vi "Setup.vi"(11 "error in":errorcluster) -> (4 "Application Ref":refnum<vi>, 6 "VI Reference Out":refnum<vi>, 15 "error out":errorcluster)   [LabVIEW 2016, in "Drona.lvlib"]
uses:
  Drona.lvlib
  _Typedefs/SetupSourceConfig.ctl
  _Typedefs/SetupEXEConfig.ctl
  GetVI/GetVIByPath.vi
  GetVI/GetVIByName.vi
  GetVI/GetVI.lvlib
  Stimulus/VI/VI.lvlib
  <vilib>/Utility/config.llb/NI_LVConfig.lvlib
  <vilib>/SLL Toolkit/SLL File IO/SLL File IO.lvlib
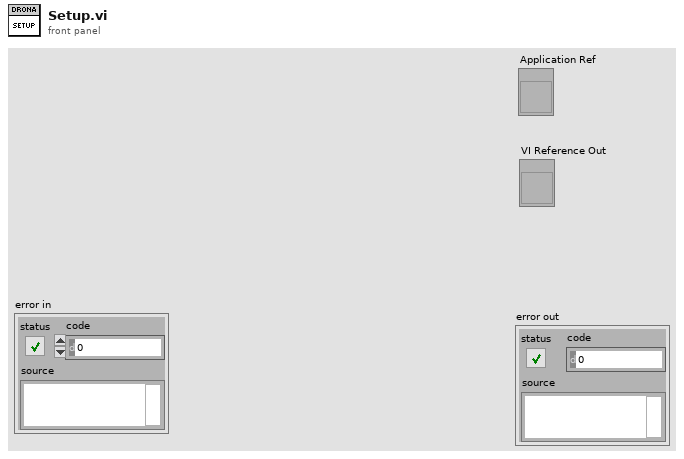
[diagram p1: front panel]
types:
  T1 = typedef "Drona.lvlib/SetupSourceConfig.ctl" = cluster{"LauncherPath":path, "Open?":bool, "Run?":bool}
  T2 = typedef "NI_LVConfig.lvlib/Config Data RefNum.ctl" = refnum<k1>
  T3 = enum32{"Bad", "Idle", "Run top level", "Running"}
  T4 = typedef "Drona.lvlib/SetupEXEConfig.ctl" = cluster{"LauncherName":string}
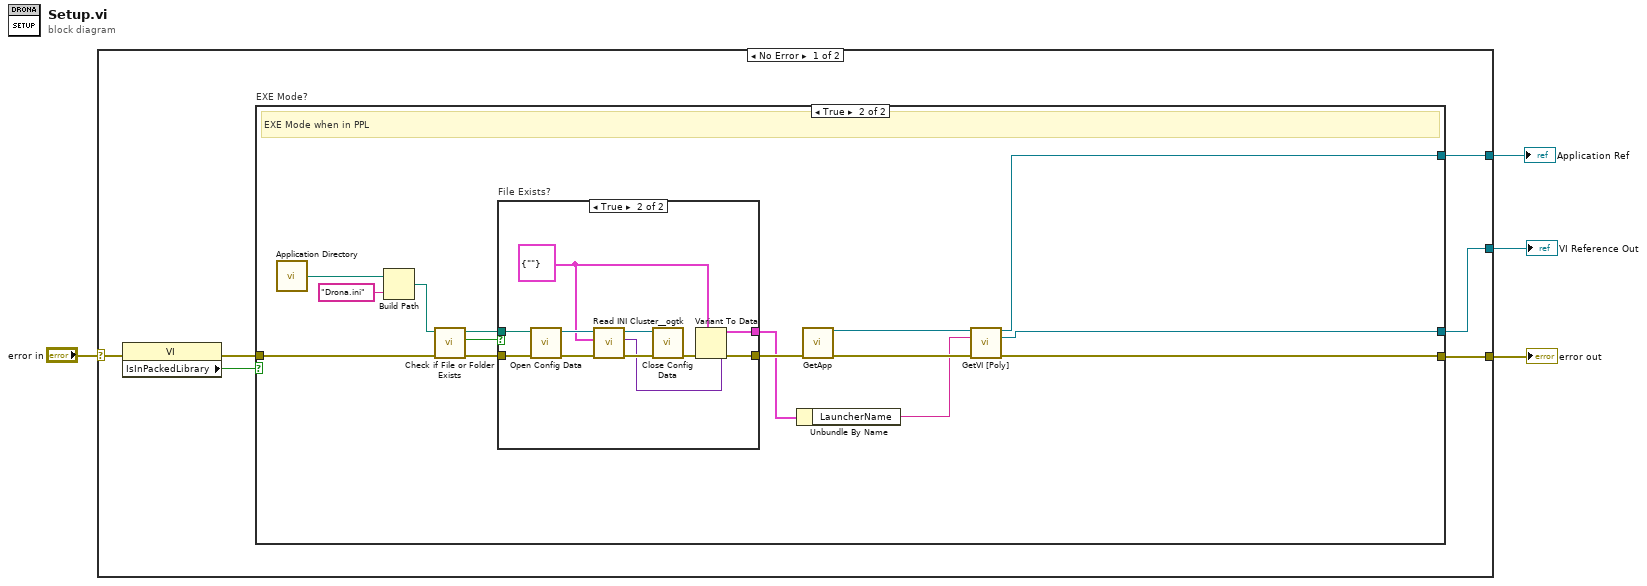
[diagram p0: block diagram]
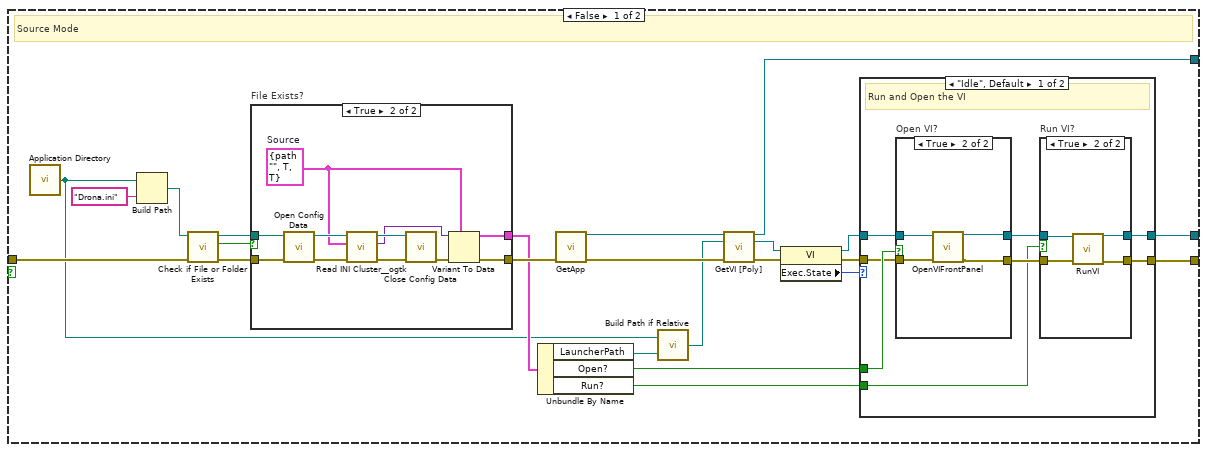
[diagram p2: hidden frame]
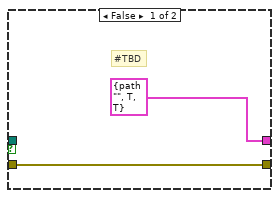
[diagram p6: hidden frame]
diagram:
  n1 = case shown="No Error" "error in" {
    selector: "error in" -> [w7 w96]
    tunnel: [w10 _] -> w3
    tunnel: [w9 _] -> w2
    tunnel: [w8 w96] -> w1
    frame No Error {
      n2 = property class="VI"(error in=w7) -> (error out=w6:errorcluster, "IsInPackedLibrary"=w5:bool)  [unwired: 1 in, 1 out]
      n3 = case "EXE Mode?" shown="True" w5 {
        tunnel: [w28 w78] -> w10
        tunnel: [w27 w77] -> w9
        tunnel: [w26 w81] -> w8
        tunnel: w6 -> [w18 w70]
        frame False {
          # "Source Mode"
          n4 = call <vilib>:"Application Directory.vi"() -> ("Application Directory"=w11:path)
          n5 = Build Path(base path=w11, name or relative path="Drona.ini") -> (appended path=w19:path)
          n6 = call <vilib>:"Check if File or Folder Exists.vi"("error in (no error)"=w18, "path"=w19) -> ("error out"=w25:errorcluster, "file or folder exists?"=w24:bool, "dup path"=w21:path)  [unwired: 7 in]
          n7 = case "File Exists?" shown="True" w24 {
            tunnel: [w57 w63] -> w30
            tunnel: [T1 {"LauncherPath"=path "", "Open?"=TRUE, "Run?"=TRUE} ("Setup Source Config") w61] -> w29
            tunnel: w25 -> [w57 w60]
            tunnel: w21 -> [_ w59]
            frame False {
              # "#TBD"
            }
            frame True {
              w58 = T1 {"LauncherPath"=path "", "Open?"=TRUE, "Run?"=TRUE}  # Source
              n8 = call <vilib>:"Open Config Data.vi"("error in (no error)"=w60, "configuration file path"=w59) -> ("error out"=w67:errorcluster, "refnum"=w66:T2)  [unwired: 7 in, 1 out]
              n9 = call <userlib>:"Read INI Cluster__ogtk.vi"("error in (no error)"=w67, "INI Fomatted Cluster Type"=w58, "refnum"=w66) -> ("error out"=w68:errorcluster, "INI Fomatted Cluster"=w62:variant, "dup refnum"=w64:T2)  [unwired: 4 in, 2 out]
              n10 = call <vilib>:"Close Config Data.vi"("error in (no error)"=w68, "refnum"=w64) -> ("error out"=w65:errorcluster)  [unwired: 8 in, 1 out]
              n11 = Variant To Data(error in=w65, type=w58, Variant=w62) -> (data=w61:T1, error out=w63:errorcluster)
            }
          }
          n12 = Unbundle By Name(w29) -> ("LauncherPath"=w13:path, "Open?"=w23:bool, "Run?"=w22:bool)
          n13 = call "GetApp.vi"("error in (no error)"=w30) -> ("Application Ref"=w32:refnum<vi>, "error out"=w33:errorcluster)  [unwired: 13 in]
          n14 = call <vilib>:"Build Path if Relative.vi"("Relative or Absolute Path"=w13, "Base Path"=w11) -> ("Path Out"=w12:path)
          n15 = call-poly "GetVI [Poly].vi"("Application Ref in"=w32, "VI Path"=w12, "error in (no error)"=w33) -> ("Application Ref out"=w28:refnum<vi>, "VI Reference"=w16:refnum<vi>, "error out"=w31:errorcluster)  [unwired: 10 in]
          n16 = property class="VI"(reference=w16, error in=w31) -> (reference out=w15:refnum<vi>, error out=w17:errorcluster, "Exec.State"=w14:T3)
          n17 = case shown="\"Idle\", Default" w14 {
            tunnel: [w39 w54] -> w27
            tunnel: [w38 w55] -> w26
            tunnel: w23 -> [w37 _]
            tunnel: w22 -> [w36 _]
            tunnel: w17 -> [w35 w55]
            tunnel: w15 -> [w34 w54]
            frame "Idle", Default {
              # "Run and Open the VI"
              n18 = case "Open VI?" shown="True" w37 {
                tunnel: [w48 w52] -> w41
                tunnel: [w49 w50] -> w40
                tunnel: w35 -> [w48 w53]
                tunnel: w34 -> [w49 w51]
                frame False {
                }
                frame True {
                  n19 = call "OpenVIFrontPanel.vi"("VI Reference In"=w51, "error in"=w53) -> ("VI Reference Out"=w50:refnum<vi>, "error out"=w52:errorcluster)  [unwired: 12 in]
                }
              }
              n20 = case "Run VI?" shown="True" w36 {
                tunnel: w41 -> [w42 w46]
                tunnel: w40 -> [w43 w47]
                tunnel: [w43 w44] -> w39
                tunnel: [w42 w45] -> w38
                frame False {
                }
                frame True {
                  n21 = call "RunVI.vi"("VI Reference In"=w47, "error in"=w46) -> ("VI Reference Out"=w44:refnum<vi>, "error out"=w45:errorcluster)  [unwired: 12 in]
                }
              }
            }
            frame "Run top level" {
              # "Already Running"
            }
          }
        }
        frame True {
          # "EXE Mode when in PPL"
          n22 = call <vilib>:"Application Directory.vi"() -> ("Application Directory"=w71:path)
          n23 = Build Path(base path=w71, name or relative path="Drona.ini") -> (appended path=w72:path)
          n24 = call <vilib>:"Check if File or Folder Exists.vi"("error in (no error)"=w70, "path"=w72) -> ("error out"=w76:errorcluster, "file or folder exists?"=w75:bool, "dup path"=w74:path)  [unwired: 7 in]
          n25 = case "File Exists?" shown="True" w75 {
            tunnel: [w84 w90] -> w80
            tunnel: [_ w88] -> w79
            tunnel: w76 -> [w84 w87]
            tunnel: w74 -> [_ w86]
            frame False {
            }
            frame True {
              w85 = T4 {"LauncherName"=""} ("EXE")
              n26 = call <vilib>:"Open Config Data.vi"("error in (no error)"=w87, "configuration file path"=w86) -> ("error out"=w94:errorcluster, "refnum"=w93:T2)  [unwired: 7 in, 1 out]
              n27 = call <userlib>:"Read INI Cluster__ogtk.vi"("error in (no error)"=w94, "INI Fomatted Cluster Type"=w85, "refnum"=w93) -> ("error out"=w95:errorcluster, "INI Fomatted Cluster"=w89:variant, "dup refnum"=w91:T2)  [unwired: 4 in, 2 out]
              n28 = call <vilib>:"Close Config Data.vi"("error in (no error)"=w95, "refnum"=w91) -> ("error out"=w92:errorcluster)  [unwired: 8 in, 1 out]
              n29 = Variant To Data(error in=w92, type=w85, Variant=w89) -> (data=w88:T4, error out=w90:errorcluster)
            }
          }
          n30 = Unbundle By Name(w79) -> ("LauncherName"=w69:string)
          n31 = call "GetApp.vi"("error in (no error)"=w80) -> ("Application Ref"=w82:refnum<vi>, "error out"=w83:errorcluster)  [unwired: 13 in]
          n32 = call-poly "GetVI [Poly].vi"("Application Ref in"=w82, "VI Name"=w69, "error in (no error)"=w83) -> ("Application Ref out"=w78:refnum<vi>, "VI Reference"=w77:refnum<vi>, "error out"=w81:errorcluster)  [unwired: 10 in]
        }
      }
    }
    frame Error {
    }
  }
  "error out" <- w1
  "VI Reference Out" <- w2
  "Application Ref" <- w3
